vi "OAT Compute Orbit Plot Output Data.vi"(6 "trigger pulse direction":u16(ring)=1 items=["positive going", "negative going"], 7 "tach duty":i32=1, 8 "actual samples/rev":dbl format="%.2f", 9 "revolutions":dbl format="%.2f", 10 "start":dbl format="%.2f", 11 "order waveform":dbl[][](array[numeric]) format="%.2f") -> (3 "orbit data":cluster{dbl[], dbl[]}[](array[cluster]) {"?" format="%.2f"; "?" format="%.2f"})   [LabVIEW 2017]
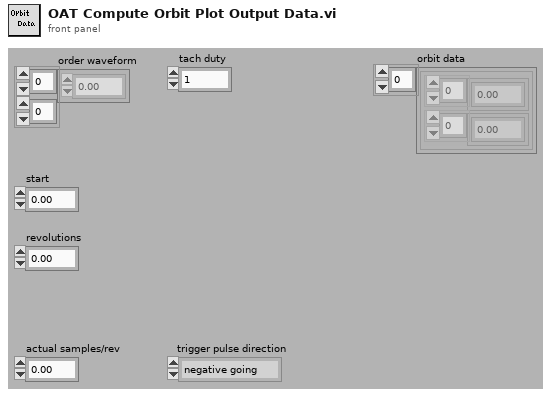
[diagram p1: front panel]
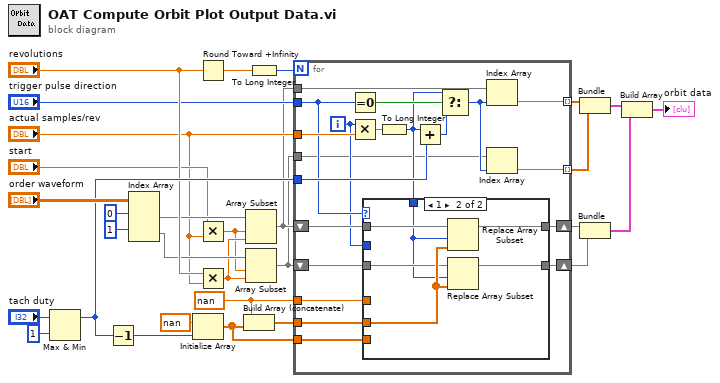
[diagram p0: block diagram]
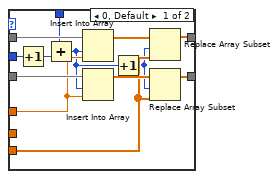
[diagram p2: hidden frame]
diagram:
  w4 = nan ("element")
  n1 = Max & Min(x="tach duty", y=1) -> (max(x,y)=w19:i32)  [unwired: 1 out]
  n2 = Decrement(x=w19) -> (x-1=w6:i32)
  n3 = Index Array(array="order waveform", index (row) #1=0 ("index (row)"), index (row) #2=1 ("index (row)")) -> (element #1=w13:dbl[], element #2=w12:dbl[])  [unwired: 2 in]
  n4 = Initialize Array(nan ("element"), w6) -> (w3:dbl[])
  n5 = Round Toward +Infinity(x="revolutions") -> (ceil(x): smallest int >= x=w20:dbl)
  n6 = Multiply(x="start", y="actual samples/rev") -> (x*y=w7:dbl)
  n7 = Multiply(x="revolutions", y="actual samples/rev") -> (x*y=w11:dbl)
  n8 = Build Array (concatenate)(w4, w3) -> (w5:dbl[])
  n9 = Array Subset(array=w13, index=w7, length=w11) -> (w2:dbl[])
  n10 = Array Subset(array=w12, index=w7, length=w11) -> (w1:dbl[])
  n11 = To Long Integer(number=w20) -> (32bit integer=w21:i32)
  n12 = for {
    N: w21 -> [_]
    tunnel: "actual samples/rev" -> [w44]
    tunnel: "trigger pulse direction" -> [w37]
    tunnel: [w50] -> w27 mode=indexing
    tunnel: [w49] -> w26 mode=indexing
    tunnel: w19 -> [w43]
    tunnel: w5 -> [w42]
    shift-right: [w40] -> w17
    shift-left: w2 -> [w41]
    shift-right: [w39] -> w16
    shift-left: w1 -> [w31]
    tunnel: w4 -> [w36]
    tunnel: w3 -> [w34]
    tunnel: w2 -> [w33]
    tunnel: w1 -> [w32]
    i -> [w35]
    n13 = Equal To 0?(x=w37) -> (x = 0?=w48:bool)
    n14 = Multiply(x=w35, y=w44) -> (x*y=w47:dbl)
    n15 = To Long Integer(number=w47) -> (32bit integer=w38:i32)
    n16 = case shown="1" w37 {
      tunnel: w42 -> [_ w69]
      tunnel: w41 -> [w63 w68]
      tunnel: [w57 w67] -> w40
      tunnel: w31 -> [w62 w66]
      tunnel: [w55 w65] -> w39
      tunnel: w38 -> [w60 w64]
      tunnel: w36 -> [w61 _]
      tunnel: w35 -> [w59 _]
      tunnel: w34 -> [w54 _]
      frame 0, Default {
        n17 = Increment(x=w59) -> (x+1=w51:i32)
        n18 = Add(x=w60, y=w51) -> (x+y=w53:i32)
        n19 = Insert Into Array(array=w63, index=w53, new element=w61) -> (w58:dbl[])
        n20 = Insert Into Array(array=w62, index=w53, new element=w61) -> (w56:dbl[])
        n21 = Increment(x=w53) -> (x+1=w52:i32)
        n22 = Replace Array Subset(array=w58, new element=w54, index=w52) -> (w57:dbl[])
        n23 = Replace Array Subset(array=w56, new element=w54, index=w52) -> (w55:dbl[])
      }
      frame 1 {
        n24 = Replace Array Subset(array=w68, new element=w69, index=w64) -> (w67:dbl[])
        n25 = Replace Array Subset(array=w66, new element=w69, index=w64) -> (w65:dbl[])
      }
    }
    n26 = Add(x=w38, y=w43) -> (x+y=w46:i32)
    n27 = Select(t=w38, s=w48, f=w46) -> (s? t:f=w45:i32)
    n28 = Index Array(array=w33, index=w45) -> (element=w50:dbl)
    n29 = Index Array(array=w32, index=w45) -> (element=w49:dbl)
  }
  n30 = Bundle(w27, w26) -> (w25:cluster{dbl[], dbl[]})  [unwired: 1 in]
  n31 = Bundle(w17, w16) -> (w15:cluster{dbl[], dbl[]})  [unwired: 1 in]
  n32 = Build Array(w25, w15) -> (→"orbit data":cluster{dbl[], dbl[]}[])
